vi "Problem 8.vi"(10 "#Adjacent Digits":i32=13, 11 "Digit String":string="7316717653133062491922511967442657474235534919493496983520312774506326239578318016984801869478851843858615607891129494954595017379583319528532088055111254069874715852386305071569329096329522744304355766896648950445244523161731856403098711121722383113622298934233803081353362766142828064444866452387493035890729629049156044077239071381051585930796086670172427121883998797908792274921901699720888093776657273330010533678812202354218097512545405947522435258490771167055601360483958644670632441572215539753697817977846174064955149290862569321978468622482839722413756570560574902614079729686524145351004748216637048440319989000889524345065854122758866688116427171479924442928230863465674813919123162824586178664583591245665294765456828489128831426076900422421902267105562632111110937054421750694165896040807198403850962455444362981230987879927244284909188845801561660979191338754992005240636899125607176060588611646710940507754100225698315520005593572972571636269561882670428252483600823257530420752963450") -> (2 "Adjacent Numbers":u64[](array[numeric]), 3 "Largest Multiple":u64)   [LabVIEW 2013, in "Problem 8.lvlib"]
uses:
  Problem 8.lvlib
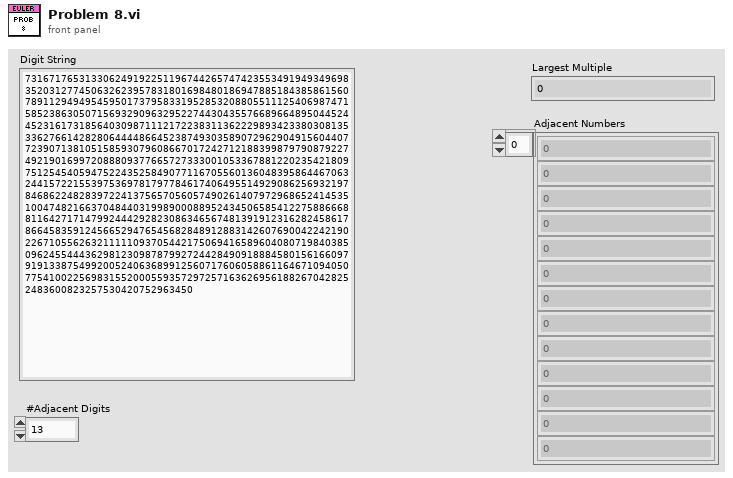
[diagram p1: front panel]
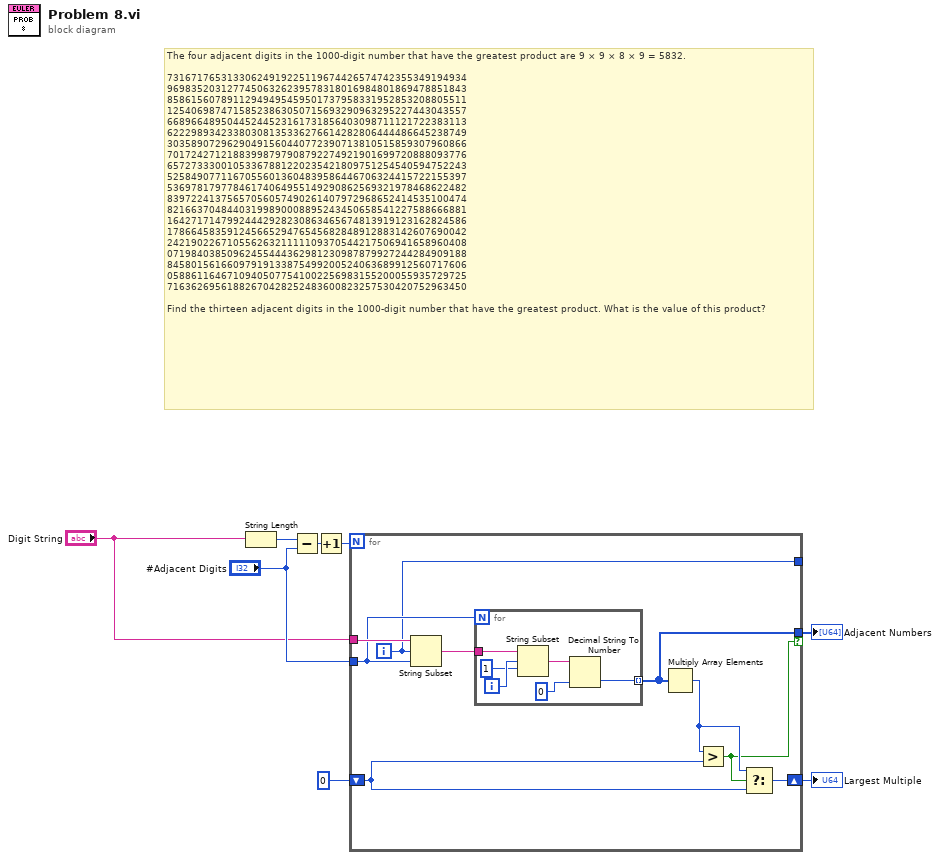
[diagram p0: block diagram]
diagram:
  # "The four adjacent digits in the 1000-digit number that have the greatest product are 9 × 9 × 8 × 9 = 5832.\n\n73167176531330624919225119674426574742355349194934\n96983520312774506326239578318016984801869478851843\n85861560789112949495459501737958331952853208805511\n12540698747158523863050715693290963295227443043557\n66896648950445244523161731856403098711121722383113\n62229893423380308135336276614282806444486645238749\n30358907296290491560440772390713810515859307960866\n70172427121883998797908792274921901699720888093776\n65727333001053367881220235421809751254540594752243\n52584907711670556013604839586446706324415722155397\n53697817977846174064955149290862569321978468622482\n83972241375657056057490261407972968652414535100474\n82166370484403199890008895243450658541227588666881\n16427171479924442928230863465674813919123162824586\n17866458359124566529476545682848912883142607690042\n24219022671055626321111109370544217506941658960408\n07198403850962455444362981230987879927244284909188\n84580156166097919133875499200524063689912560717606\n05886116467109405077541002256983155200055935729725\n71636269561882670428252483600823257530420752963450\n\nFind the thirteen adjacent digits in the 1000-digit number that have the greatest product. What is the value of this product?"
  n1 = String Length(string="Digit String") -> (length=w8:i32)
  n2 = Subtract(x=w8, y="#Adjacent Digits") -> (x-y=w7:i32)
  n3 = Increment(x=w7) -> (x+1=w4:i32)
  n4 = for {
    N: w4 -> [_]
    tunnel: "Digit String" -> [w17]
    tunnel: "#Adjacent Digits" -> [w15]
    shift-right: [w12] -> w1
    shift-left: u64 0 -> [w13]
    tunnel: [w11] -> w2 if=w10
    tunnel: [w9] -> _
    i -> [w9]
    n5 = String Subset(string=w17, offset (0)=w9, length (rest)=w15) -> (substring=w16:string)
    n6 = for {
      N: w15 -> [_]
      tunnel: w16 -> [w23]
      tunnel: [w19] -> w11 mode=indexing
      i -> [w22]
      n7 = String Subset(string=w23, offset (0)=w22, length (rest)=1 ("length (rest)")) -> (substring=w20:string)
      n8 = Decimal String To Number(string=w20, default (0L)=u64 0) -> (number=w19:u64)  [unwired: 1 in, 1 out]
    }
    n9 = Multiply Array Elements(1:w11) -> (0:w14:u64)
    n10 = Greater?(x=w14, y=w13) -> (0:w10:bool)
    n11 = Select(t=w14, s=w10, f=w13) -> (s? t:f=w12:u64)
  }
  "Adjacent Numbers" <- w2
  "Largest Multiple" <- w1
